vi "Assorted Calculation.vi"() -> ()   [LabVIEW 2020]
panel:
  out "y":dbl
  out "x":dbl
  out "Conductance":cdb
  out "|Z|":dbl
  out "Impedance":cdb
  out "START":cdb
  out "loss db":dbl
  out "degree":dbl
  out "Magnitude":dbl
  out "theta":dbl
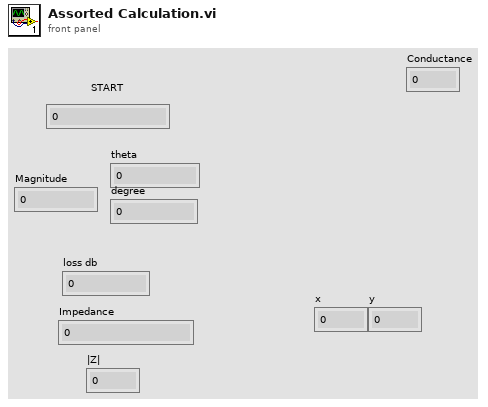
[diagram p1: front panel]
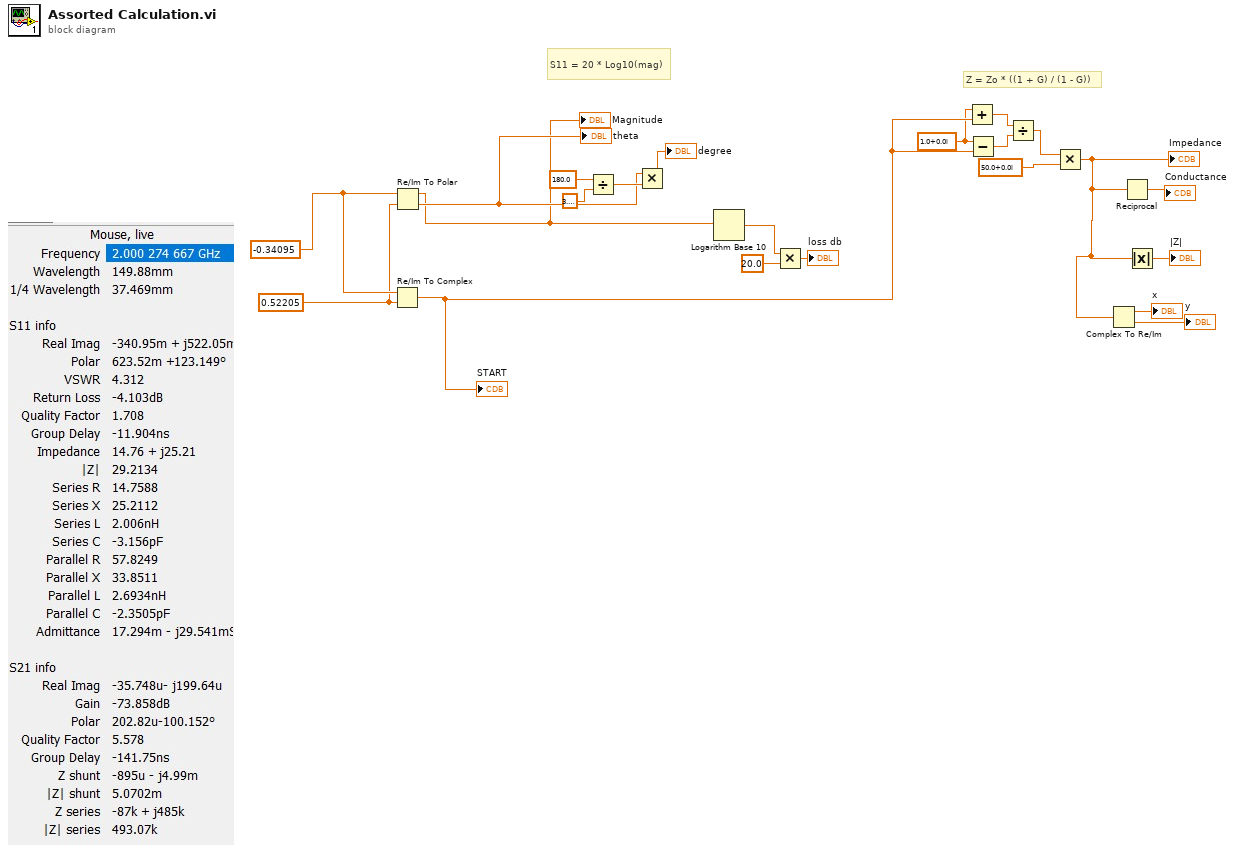
[diagram p0: block diagram]
diagram:
  w10 = cdb 1.0+0.0i ("x")
  w14 = 0.52205 ("x")
  w15 = -0.34095 ("x")
  # "Z = Zo * ((1 + G) / (1 - G))"
  # "S11 = 20 * Log10(mag)"
  n1 = Re/Im To Complex(1:w14, 2:w15) -> (0:w11:cdb)
  "START" <- w11
  n2 = Re/Im To Polar(2:w14, 3:w15) -> (0:w13:dbl, 1:w12:dbl)
  "theta" <- w13
  "Magnitude" <- w12
  n3 = Divide(x=180.0, y=3.141592653589793) -> (x/y=w20:dbl)
  n4 = Multiply(x=w13, y=w20) -> (x*y=→"degree":dbl)
  n5 = Logarithm Base 10(1:w12) -> (0:w18:dbl)
  n6 = Multiply(x=w18, y=20.0) -> (x*y=→"loss db":dbl)
  n7 = Add(x=w10, y=w11) -> (x+y=w9:cdb)
  n8 = Subtract(x=w10, y=w11) -> (x-y=w8:cdb)
  n9 = Divide(x=w9, y=w8) -> (x/y=w7:cdb)
  n10 = Multiply(x=w7, y=cdb 50.0+0.0i) -> (x*y=w3:cdb)
  "Impedance" <- w3
  n11 = Complex To Re/Im(x + iy=w3) -> (x=→"x":dbl, y=→"y":dbl)
  n12 = Reciprocal(x=w3) -> (1/x=→"Conductance":cdb)
  n13 = Absolute Value(x=w3) -> (abs(x)=→"|Z|":dbl)
